vi "aft_FXP_LMS_X_Address_Generator.vi"(7 "first run? (F)":bool, 10 "filter length":u32, 11 "state in":u32) -> (3 "state out":u32)   [LabVIEW 2017]
doc: "This VI generates addresses for reading x(n) from RAM."
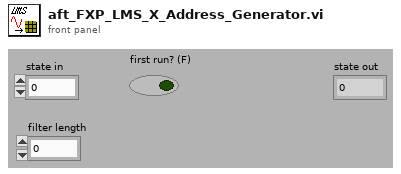
[diagram p1: front panel]
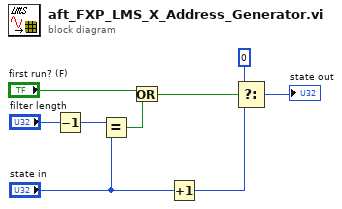
[diagram p0: block diagram]
diagram:
  n1 = Decrement(x="filter length") -> (x-1=w2:u32)
  n2 = Equal?(x=w2, y="state in") -> (x = y?=w6:bool)
  n3 = Or(x="first run? (F)", y=w6) -> (x .or. y?=w3:bool)
  n4 = Increment(x="state in") -> (x+1=w4:u32)
  n5 = Select(t=u32 0, s=w3, f=w4) -> (s? t:f=→"state out":u32)
